vi "#30_MAV_MSG_ATTITUDE.vi"(11 "mavlink_payload":u8[](array[numeric])) -> (3 "ATTITUDE":T1)   [LabVIEW 2023]
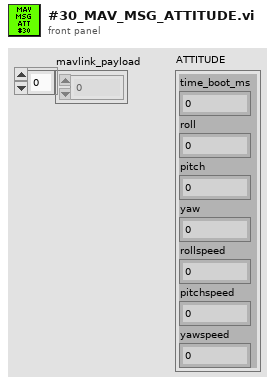
[diagram p1: front panel]
types:
  T1 = cluster{"time_boot_ms":u32, "roll":sgl, "pitch":sgl, "yaw":sgl, "rollspeed":sgl, "pitchspeed":sgl, "yawspeed":sgl}
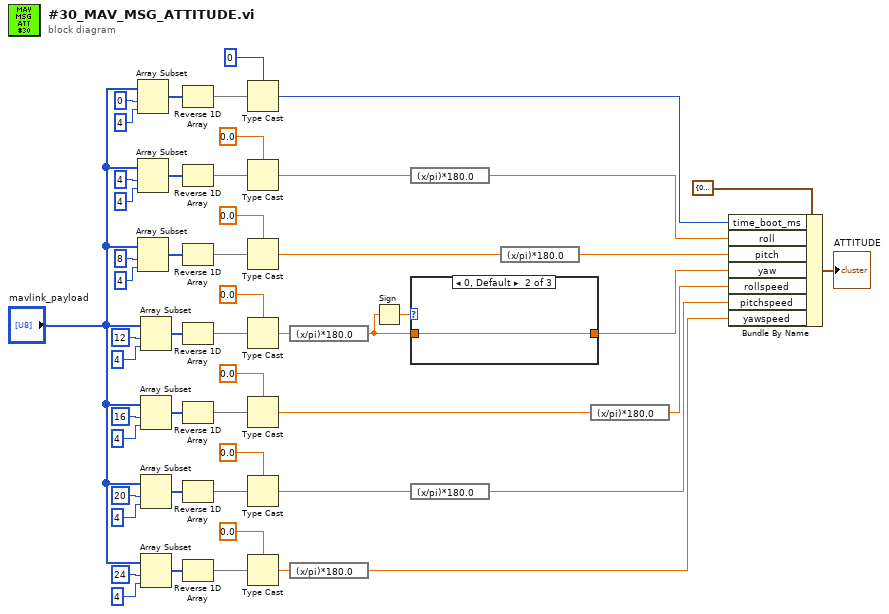
[diagram p0: block diagram]
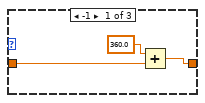
[diagram p2: hidden frame]
diagram:
  n1 = Array Subset(array="mavlink_payload", index=0, length=4) -> (w53:u8[])
  n2 = Array Subset(array="mavlink_payload", index=4, length=4) -> (w45:u8[])
  n3 = Array Subset(array="mavlink_payload", index=8, length=4) -> (w40:u8[])
  n4 = Array Subset(array="mavlink_payload", index=12, length=4) -> (w35:u8[])
  n5 = Array Subset(array="mavlink_payload", index=16, length=4) -> (w30:u8[])
  n6 = Array Subset(array="mavlink_payload", index=20, length=4) -> (w25:u8[])
  n7 = Array Subset(array="mavlink_payload", index=24, length=4) -> (w20:u8[])
  n8 = Reverse 1D Array(array=w53) -> (reversed array=w52:u8[])
  n9 = Reverse 1D Array(array=w45) -> (reversed array=w44:u8[])
  n10 = Reverse 1D Array(array=w40) -> (reversed array=w39:u8[])
  n11 = Reverse 1D Array(array=w35) -> (reversed array=w34:u8[])
  n12 = Reverse 1D Array(array=w30) -> (reversed array=w29:u8[])
  n13 = Reverse 1D Array(array=w25) -> (reversed array=w24:u8[])
  n14 = Reverse 1D Array(array=w20) -> (reversed array=w19:u8[])
  n15 = Type Cast(type=u32 0 ("single precision float"), x=w52) -> (*(type *) &x=w47:u32)
  n16 = Type Cast(type=sgl 0.0 ("single precision float"), x=w44) -> (*(type *) &x=w12:sgl)
  n17 = Type Cast(type=sgl 0.0 ("single precision float"), x=w39) -> (*(type *) &x=w11:sgl)
  n18 = Type Cast(type=sgl 0.0 ("single precision float"), x=w34) -> (*(type *) &x=w13:sgl)
  n19 = Type Cast(type=sgl 0.0 ("single precision float"), x=w29) -> (*(type *) &x=w8:sgl)
  n20 = Type Cast(type=sgl 0.0 ("single precision float"), x=w24) -> (*(type *) &x=w7:sgl)
  n21 = Type Cast(type=sgl 0.0 ("single precision float"), x=w19) -> (*(type *) &x=w14:sgl)
  n22 = expression code="(x/pi)*180.0" ("radians to degrees")(w13) -> (w2:sgl)
  n23 = expression code="(x/pi)*180.0" ("radians to degrees")(w14) -> (w6:sgl)
  n24 = Sign(1:w2) -> (0:w3:sgl)
  n25 = expression code="(x/pi)*180.0" ("radians to degrees")(w12) -> (w10:sgl)
  n26 = case shown="0, Default" w3 {
    tunnel: w2 -> [w55 w57 w58]
    tunnel: [w54 w57 w58] -> w1
    frame -1 {
      n27 = Add(x=sgl 360.0, y=w55) -> (x+y=w54:sgl)
    }
    frame 0, Default {
    }
    frame 1 {
    }
  }
  n28 = expression code="(x/pi)*180.0" ("radians to degrees")(w7) -> (w4:sgl)
  n29 = expression code="(x/pi)*180.0" ("radians to degrees")(w11) -> (w9:sgl)
  n30 = expression code="(x/pi)*180.0" ("radians to degrees")(w8) -> (w5:sgl)
  n31 = Bundle By Name(cluster=T1 {"time_boot_ms"=0, "roll"=0.0, "pitch"=0.0, "yaw"=0.0, "rollspeed"=0.0, "pitchspeed"=0.0, "yawspeed"=0.0} ("ATTITUDE"), "time_boot_ms"=w47, "roll"=w10, "pitch"=w9, "yaw"=w1, "rollspeed"=w5, "pitchspeed"=w4, "yawspeed"=w6) -> (→"ATTITUDE":T1)
